vi "test stim.vi"() -> ()   [LabVIEW 2010]
uses:
  <vilib>/userDefined/High Color/nirio_resource_hc.ctl
  <vilib>/Platform/TimedLoop/XDataNode/XDataNode.xnode
  <vilib>/Platform/TimedLoop/XDataNode/timing_clust.ctl
  <vilib>/Platform/TimedLoop/XDataNode/nitl_modes.ctl
  <vilib>/Platform/TimedLoop/XDataNode/wakeup.ctl
  <vilib>/rvi/interface/nirviOpenFPGA/nirviOpenFPGA.xnode
  main.lvbitx
  <vilib>/rvi/ClientSDK/nirviWhatTheDeviceIsDoing.ctl
  <vilib>/rvi/interface/nirviMethod/nirviMethod.xnode
  <vilib>/rvi/interface/common/niFpgaNodeNameForErrorReporting.ctl
  <vilib>/rvi/errors/niLvFpgaWhatHappensToTopLevelVI.ctl
  <vilib>/rvi/interface/nirviReadWriteControl/nirviReadWriteControl.xnode
  <vilib>/FPGAPlugInAG/PCIe-7842R/niLvFpga_Open_PCIe-7842R.vi
  <vilib>/rvi/interface/common/dynamic/niFpgaDynamicAddResources.vi
  <vilib>/FPGAPlugInAG/Dynamic/niLvFpga_Reset_Dynamic.vi
  <vilib>/Utility/error.llb/Error Cluster From Error Code.vi
  <vilib>/rvi/errors/niLvFpgaAdjustHostInterfaceError.vi
  <vilib>/Utility/file.llb/Write To Spreadsheet File (DBL).vi
  NiFpgaLv.dll
  <vilib>/Platform/TimedLoop/XDataNode/XDNodeRunTimeDep.lvlib
panel:
  out "counter":u16
  out "hs divisor":u8
  out "set time per sweep":dbl format="%#_6p"
  out "time per sweep":dbl format="%#_6p"
  out "total counting time":dbl
  out "ratio":cluster{dbl[], dbl[]}(graph)
  out "stop 2":bool
  out "host data":u32[](array[numeric])
  in  "count time (ns)":dbl=25.0 min=25.0 step=25.0
  in  "save":bool
  out "rate1":dbl[](array[numeric])
  out "rate0":dbl[](array[numeric])
  out "time":dbl[](array[numeric])
  in  "stim delay":u16
  out "elements queued in fifo":u32
  out "Timed Out?":bool
  out "photons sent loop2loop":u32
  out "ch0 photons loop2loop":u32
  out "ch0 photons received":u32
  out "ch0 photons sent":u32
  out "total photons ch0":u32
  in  "stop":bool
  out "count rates":cluster{dbl[], dbl[]}[](graph)
  out "data buffer length":u32
  out "sweeps counted":u32
  in  "stim enable":bool
  in  "stim counts":u16=24
  in  "count photons":bool
  in  "cycle width":u16=500 max=45000
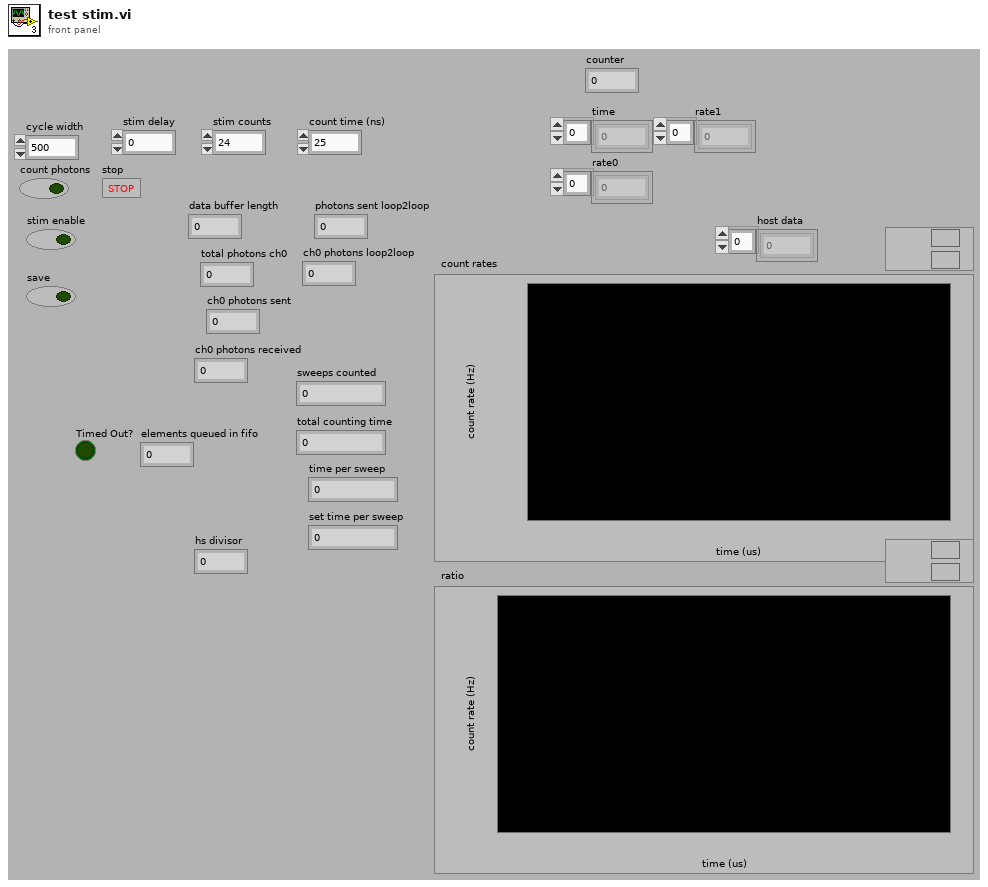
[diagram p1: front panel]
types:
  T1 = typedef "nirio_resource_hc.ctl" = tag
  T2 = typedef "XDNodeRunTimeDep.lvlib/timing_clust.ctl" = cluster{"Expected End [f-1]":u64, "Actual End [f-1]":u64, "Finished Late? [f-1]":bool, "Expected End [i-1]":u64, "Actual End [i-1]":u64, "Finished Late? [i-1]":bool, "Expected Start [i]":u64, "Actual Start [i]":u64, "Expected Start [f]":u64, "Actual Start [f]":u64, "Source Name":string, "Structure Name":string, "Period":i64, "Deadline":i64, "Offset":i64, "Start":i64, "Priority":i32, "Timeout":i32, "Mode":T3, "Wakeup Reason":T4, "Error":errorcluster, "Source Type":string, "Secondary Source Type":string, "Global End Time":u64, "Global Start Time":u64, "Frame Duration":u64, "Iteration Duration":u64, "Assigned CPU":i32, "I/O Scan Engine Mode":u32}
  T3 = typedef "XDNodeRunTimeDep.lvlib/nitl_modes.ctl" = enum32{"No Change", "Process missed periods, maintain original phase", "Discard missed periods, maintain original phase", "Process missed periods, ignore original phase", "Discard missed periods, ignore original phase"}
  T4 = typedef "XDNodeRunTimeDep.lvlib/wakeup.ctl" = enum32{"Normal", "Aborted", "Asynchronous wakeup", "Timing source error", "Timed loop error", "Timeout"}
  T5 = typedef "niFpgaNodeNameForErrorReporting.ctl" = enum16{"Open FPGA VI Reference", "Read/Write Control", "Invoke Method: Abort", "Invoke Method: Acknowledge IRQ", "Invoke Method: Download", "Invoke Method: FIFO.Configure", "Invoke Method: FIFO.Read", "Invoke Method: FIFO.Start", "Invoke Method: FIFO.Stop", "Invoke Method: FIFO.Write", "Invoke Method: Reset", "Invoke Method: Run", "Invoke Method: Wait on IRQ", "Close FPGA VI Reference"}
  T6 = typedef "niLvFpgaWhatHappensToTopLevelVI.ctl" = enum16{"top level VI scripted behind XNode", "top level VI inlined behind XNode"}
  T7 = typedef "imagedata.ctl" = cluster{"image type":i32, "image depth":i32, "image":u8[], "mask":u8[], "colors":u32[], "Rectangle":cluster{"left":i16, "top":i16, "right":i16, "bottom":i16}}
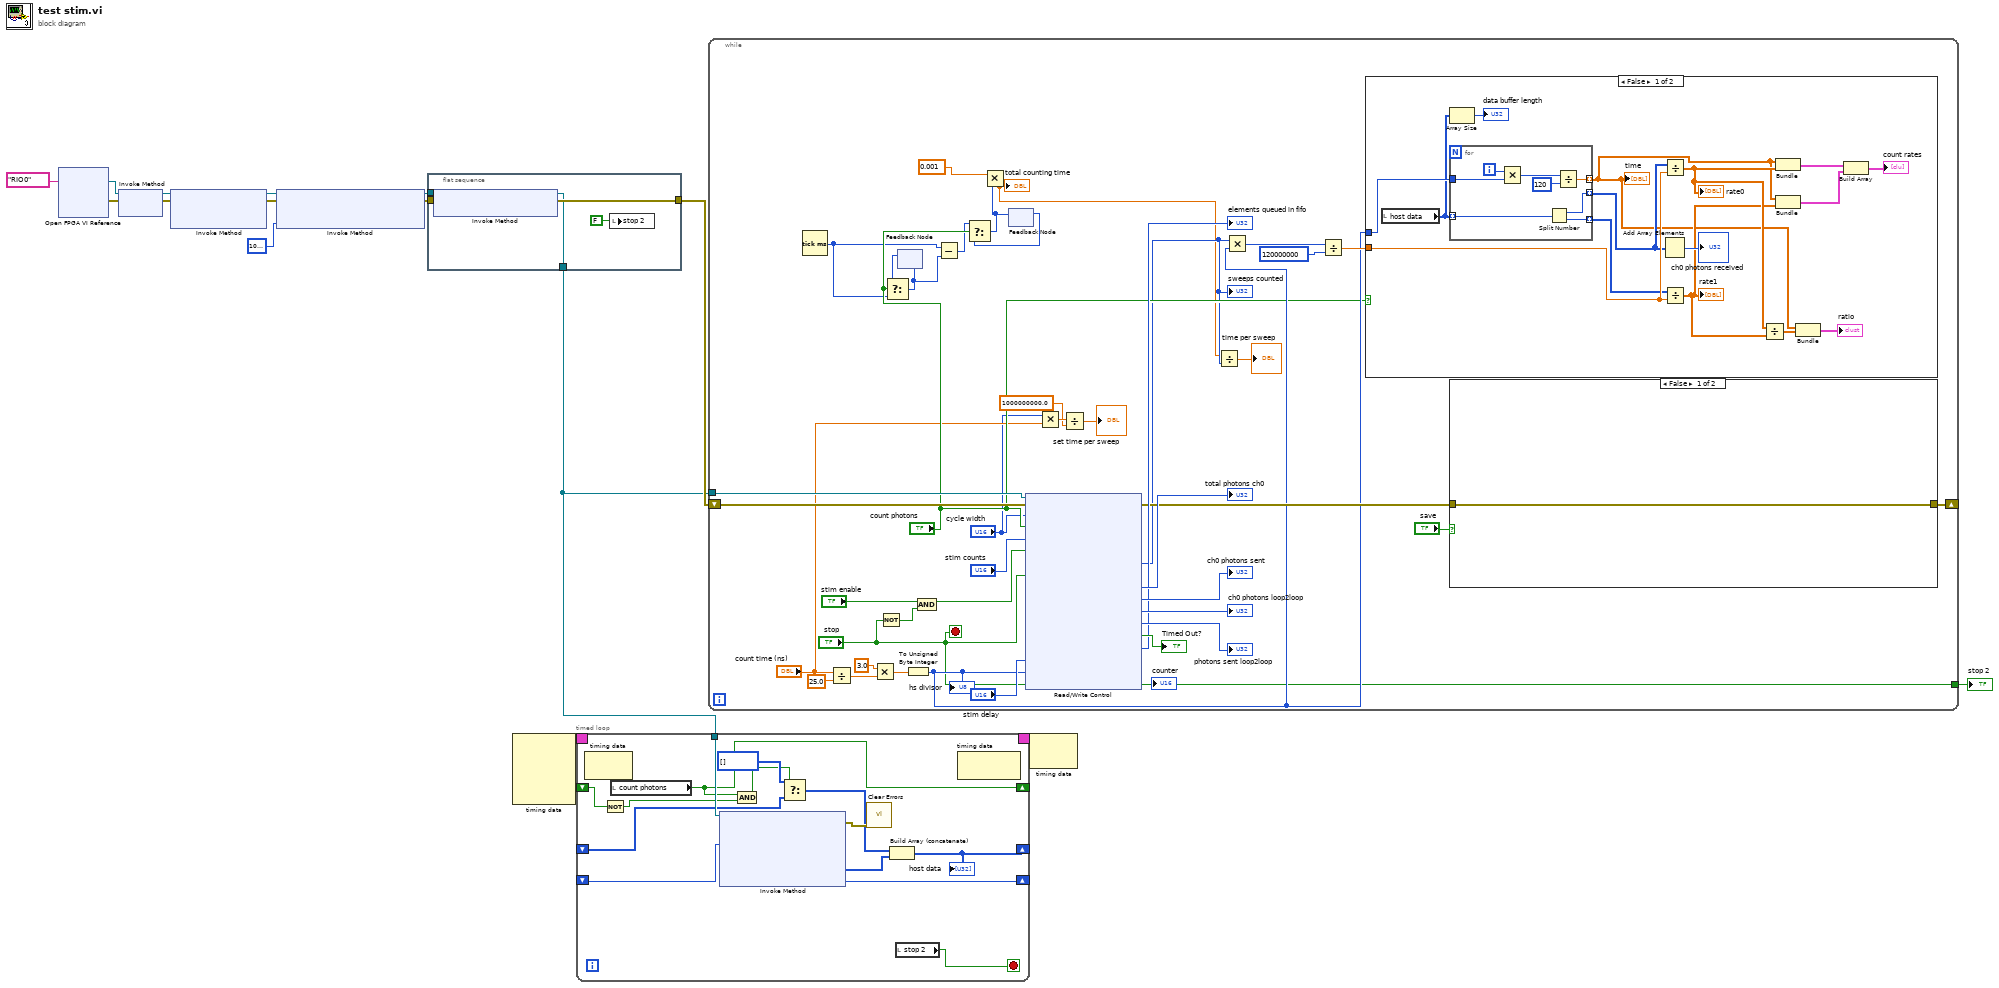
[diagram p0: block diagram]
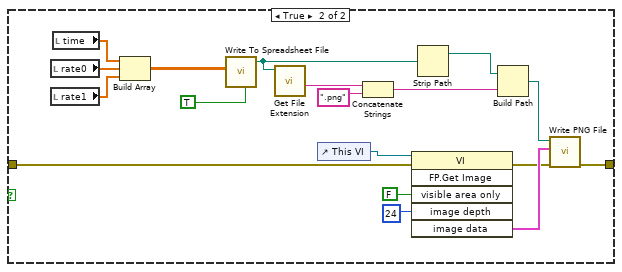
[diagram p2: hidden frame]
diagram:
  n1 = xnode "Open FPGA VI Reference"("resource name"=T1 "RIO0") -> ("FPGA VI Reference Out"=w10:refnum<k20>, "error out"=w9:errorcluster)  [unwired: 1 in]
  n2 = xnode "Invoke Method"("FPGA VI Reference In"=w10, "error in"=w9) -> ("FPGA VI Reference Out"=w8:refnum<k20>, "error out"=w7:errorcluster)
  n3 = xnode "Invoke Method"("FPGA VI Reference In"=w8, "error in"=w7) -> ("FPGA VI Reference Out"=w6:refnum<k20>, "error out"=w5:errorcluster)  [unwired: 1 in]
  n4 = xnode "Invoke Method"("FPGA VI Reference In"=w6, "error in"=w5, "Depth"=u32 1000000) -> ("FPGA VI Reference Out"=w13:refnum<k20>, "error out"=w12:errorcluster)
  n5 = flat-sequence {
    tunnel: w13 -> [w20]
    tunnel: w12 -> [w19]
    tunnel: [w18] -> w11
    tunnel: [w17] -> w2
    frame #0 {
      n6 = xnode "Invoke Method"("FPGA VI Reference In"=w20, "error in"=w19) -> ("FPGA VI Reference Out"=w17:refnum<k20>, "error out"=w18:errorcluster)
      n7 = local write "stop 2"(FALSE ("stop 2")) -> ()
    }
  }
  n8 = node-c288() -> (w4:T2)  [unwired: 4 in]
  n9 = timed-loop {
    timing: w4 -> [_]
    timing-out: [_] -> w3
    shift-right: [w56] -> _
    shift-left: _ -> [w55]
    tunnel: w2 -> [w54]
    shift-right: [w51] -> _
    shift-left: _ -> [w49]
    shift-right: [w46] -> _
    shift-left: _ -> [w45]
    stop <- w43 stop-if-true
    n10 = node-c288() -> ()  [unwired: 1 in, 1 out]
    n11 = Not(x=w45) -> (.not. x?=w44:bool)
    n12 = local read "count photons"() -> (w46:bool)
    n13 = xnode "Invoke Method"("FPGA VI Reference In"=w54, "Number of Elements"=w55) -> ("error out"=w53:errorcluster, "Data"=w52:u32[], "Elements Remaining"=w56:u32)  [unwired: 2 in, 1 out]
    n14 = And(x=w46, y=w44) -> (x .and. y?=w47:bool)
    n15 = Select(t=u32[] [], s=w47, f=w49) -> (s? t:f=w48:u32[])
    n16 = call <vilib>:"Clear Errors.vi"("error in (no error)"=w53) -> ()  [unwired: 6 in, 1 out]
    n17 = Build Array (concatenate)(w48, w52) -> (w51:u32[])
    "host data" <- w51
    n18 = local read "stop 2"() -> (w43:bool)
    n19 = node-c288() -> ()  [unwired: 1 in, 1 out]
  }
  n20 = while {
    tunnel: w2 -> [w173]
    shift-right: [w158] -> _
    shift-left: w11 -> [w170]
    tunnel: ["stop"] -> w1
    stop <- "stop" stop-if-true
    n21 = Tick Count (ms)() -> (millisecond timer value=w144:u32)
    n22 = Divide(x="count time (ns)", y=25.0) -> (x/y=w156:dbl)
    n23 = Multiply(x=3.0, y=w156) -> (x*y=w154:dbl)
    n24 = Not(x="stop") -> (.not. x?=w150:bool)
    n25 = feedback #1() -> (w143:u32)  [unwired: 1 in]
    n26 = Select(t=w143, s="count photons", f=w144) -> (s? t:f=w147:u32)
    n27 = feedback-in #1(w147) -> ()
    n28 = To Unsigned Byte Integer(number=w154) -> (unsigned 8bit integer=w152:u8)
    "hs divisor" <- w152
    n29 = And(x="stim enable", y=w150) -> (x .and. y?=w151:bool)
    n30 = Subtract(x=w144, y=w147) -> (x-y=w146:u32)
    n31 = feedback #2() -> (w145:u32)  [unwired: 1 in]
    n32 = Select(t=w146, s="count photons", f=w145) -> (s? t:f=w135:u32)
    n33 = Multiply(x=0.001, y=w135) -> (x*y=w134:dbl)
    "total counting time" <- w134
    n34 = feedback-in #2(w135) -> ()
    n35 = xnode "Read/Write Control"("FPGA VI Reference In"=w173, "error in"=w170, "cycle width"="cycle width", "count photons"="count photons", "stim counts"="stim counts", "stim enable"=w151, "stop"="stop", "stim delay"="stim delay", "HS divisor"=w152) -> ("error out"=w159:errorcluster, "sweeps counted"=w142:u32, "total photons ch0"=→"total photons ch0":u32, "ch0 photons sent"=→"ch0 photons sent":u32, "ch0 photons loop2loop"=→"ch0 photons loop2loop":u32, "photons sent loop2loop"=→"photons sent loop2loop":u32, "Timed Out?"=→"Timed Out?":bool, "elements queued in fifo"=→"elements queued in fifo":u32, "counter"=→"counter":u16)  [unwired: 1 out]
    "sweeps counted" <- w142
    n36 = Multiply(x="cycle width", y="count time (ns)") -> (x*y=w138:dbl)
    n37 = Divide(x=w138, y=1000000000.0) -> (x/y=→"set time per sweep":dbl)
    n38 = Divide(x=w134, y=w142) -> (x/y=→"time per sweep":dbl)
    n39 = Multiply(x=w142, y=w152) -> (x*y=w153:u32)
    n40 = Divide(x=w153, y=u32 120000000) -> (x/y=w168:dbl)
    n41 = case shown="False" "count photons" {
      tunnel: w168 -> [w205 _]
      tunnel: w152 -> [w201 _]
      frame False {
        n42 = local read "host data"() -> (w200:u32[])
        n43 = Array Size(array=w200) -> (size(s)=→"data buffer length":i32)
        n44 = for {
          tunnel: [w212] -> w193 mode=indexing
          tunnel: [w214] -> w204 mode=indexing
          tunnel: [w213] -> w195 mode=indexing
          tunnel: w201 -> [w209]
          tunnel: w200 -> [w208] mode=indexing
          i -> [w215]
          n45 = Multiply(x=w215, y=w209) -> (x*y=w210:i32)
          n46 = Split Number(x=w208) -> (hi(x)=w214:u16, lo(x)=w213:u16)
          n47 = Divide(x=w210, y=120) -> (x/y=w212:dbl)
        }
        "time" <- w193
        n48 = Add Array Elements(numeric array=w204) -> (sum=→"ch0 photons received":u16)
        n49 = Divide(x=w204, y=w205) -> (x/y=w198:dbl[])
        "rate0" <- w198
        n50 = Divide(x=w195, y=w205) -> (x/y=w197:dbl[])
        "rate1" <- w197
        n51 = Divide(x=w198, y=w197) -> (x/y=w196:dbl[])
        n52 = Bundle(w193, w198) -> (w207:cluster{dbl[], dbl[]})  [unwired: 1 in]
        n53 = Bundle(w193, w197) -> (w202:cluster{dbl[], dbl[]})  [unwired: 1 in]
        n54 = Bundle(w193, w196) -> (→"ratio":cluster{dbl[], dbl[]})  [unwired: 1 in]
        n55 = Build Array(w207, w202) -> (→"count rates":cluster{dbl[], dbl[]}[])
      }
      frame True {
      }
    }
    n56 = case shown="False" "save" {
      tunnel: [w174 w177] -> w158
      tunnel: w159 -> [w174 w176]
      frame False {
      }
      frame True {
        n57 = local read "rate0"() -> (w191:dbl[])
        n58 = local read "rate1"() -> (w190:dbl[])
        n59 = local read "time"() -> (w192:dbl[])
        n60 = Build Array(w192, w191, w190) -> (w189:dbl[][])
        n61 = call-poly <vilib>:"Write To Spreadsheet File.vi"("transpose? (no:F)"=TRUE, "2D data"=w189) -> ("new file path (Not A Path if cancelled)"=w188:path)  [unwired: 6 in]
        n62 = call <vilib>:"Get File Extension.vi"("file"=w188) -> ("filename without extension"=w185:string)  [unwired: 7 in, 3 out]
        n63 = control-ref of="This VI"() -> (w187:refnum<vi>)
        n64 = Concatenate Strings(w185, ".png" ("string")) -> (w183:string)
        n65 = invoke class="VI" method="FP.Get Image"(reference=w187, error in=w176, "visible area only"=FALSE ("Visible Area Only"), "image depth"=24 ("Image Depth")) -> (error out=w179:errorcluster, "image data"=w180:T7)  [unwired: 2 in, 4 out]
        n66 = Strip Path(path=w188) -> (stripped path=w182:path)  [unwired: 1 out]
        n67 = Build Path(base path=w182, name or relative path=w183) -> (appended path=w181:path)
        n68 = call <vilib>:"Write PNG File.vi"("error in (no error)"=w179, "image data"=w180, "path to PNG file"=w181) -> ("error out"=w177:errorcluster)  [unwired: 7 in, 1 out]
      }
    }
  }
  "stop 2" <- w1
  n69 = node-c288(w3) -> ()  [unwired: 1 out]
